vi "Periodic Tasks.vi"(8 "error in":errorcluster) -> ()   [LabVIEW 2023]
doc: "This VI runs in parallel to other tasks. It can contain as many user-defined periodic loops as you need. These can carry out PID or other sorts of timed response."
uses:
  Global odometry.vi
  Global INIT.vi
  <vilib>/Analysis/NI_AAL_Angle.lvlib
  <vilib>/Analysis/coordinate.llb/Wrap Angle (scalar).vi
  <vilib>/Analysis/coordinate.llb/Angle Units.ctl
  <vilib>/Analysis/coordinate.llb/Angle Range (Degree).ctl
  ctrl defs/ctrl DRIVER target assist.ctl
  <vilib>/Rock Robotics/WPI/DriverStation/WPI_DriverStationAllianceInfo.ctl
  ctrl defs/ctrl DRIVING FRAME selector.ctl
  ctrl defs/ctrl pivot select.ctl
  ctrl defs/ctrl driver input.ctl
  ctrl defs/ctrl FRONT FACE selector.ctl
  ctrl defs/ctrl XY coord.ctl
  ctrl defs/ctrl LIMELIGHT STREAM selector.ctl
  ctrl defs/ctrl LIMELIGHT CAMMODE selector.ctl
  ctrl defs/ctrl LIMELIGHT LEDMODE selector.ctl
panel:
  out "LimeLIGHT control":T4 {"stream" items=["standard side-by-side", "PiP Main", "PiP Secondary"]; "camMode" items=["Vision processor", "Driver Camera"]; "ledMode" items=["default to current pipeline", "force off", "force blink", "force on"]}
  out "DRIVER TARGET ASSIST":T5={"ASSIST?"=FALSE, "LOCKED ON?"=FALSE, "DistanceToTarget (in)"=26.235051697949295, "BRNG (deg)"=-2.0}
  out "Continuous Angle":T6
  in  "Update":bool
  out "pivot center":T7 {"Y" format="%.4g"; "X" format="%.4g"}
  out "front face":T8
  out "DRIVER INPUT":T9 {"Jr" format="%.4g"; "theta (rad)" format="%_4f"; "R" format="%.4g"; "Jy" format="%.4g"; "theta (deg)" format="%_4f"; "Jx" format="%.4g"}
  out "select pivot point":T10
  out "drive frame":T11
  out "Alliance":T12
  out "STEER":dbl
  out "DRIVE":dbl
  out "YRPHfH":T13
  out "REAR RIGHT":dbl(knob)
  out "V RR":dbl(knob) scale=-1.0..1.0
  out "FRONT RIGHT":dbl(knob)
  out "V FR":dbl(knob) scale=-1.0..1.0
  out "REAR LEFT":dbl(knob)
  out "V RL":dbl(knob) scale=-1.0..1.0
  out "FRONT LEFT":dbl(knob)
  out "V FL":dbl(knob) scale=-1.0..1.0
  out "Magnetic\nHeadings":cluster{dbl, dbl, dbl}(knob)={0.0, 140.19422999815168, 0.0} scale=0.0..360.0
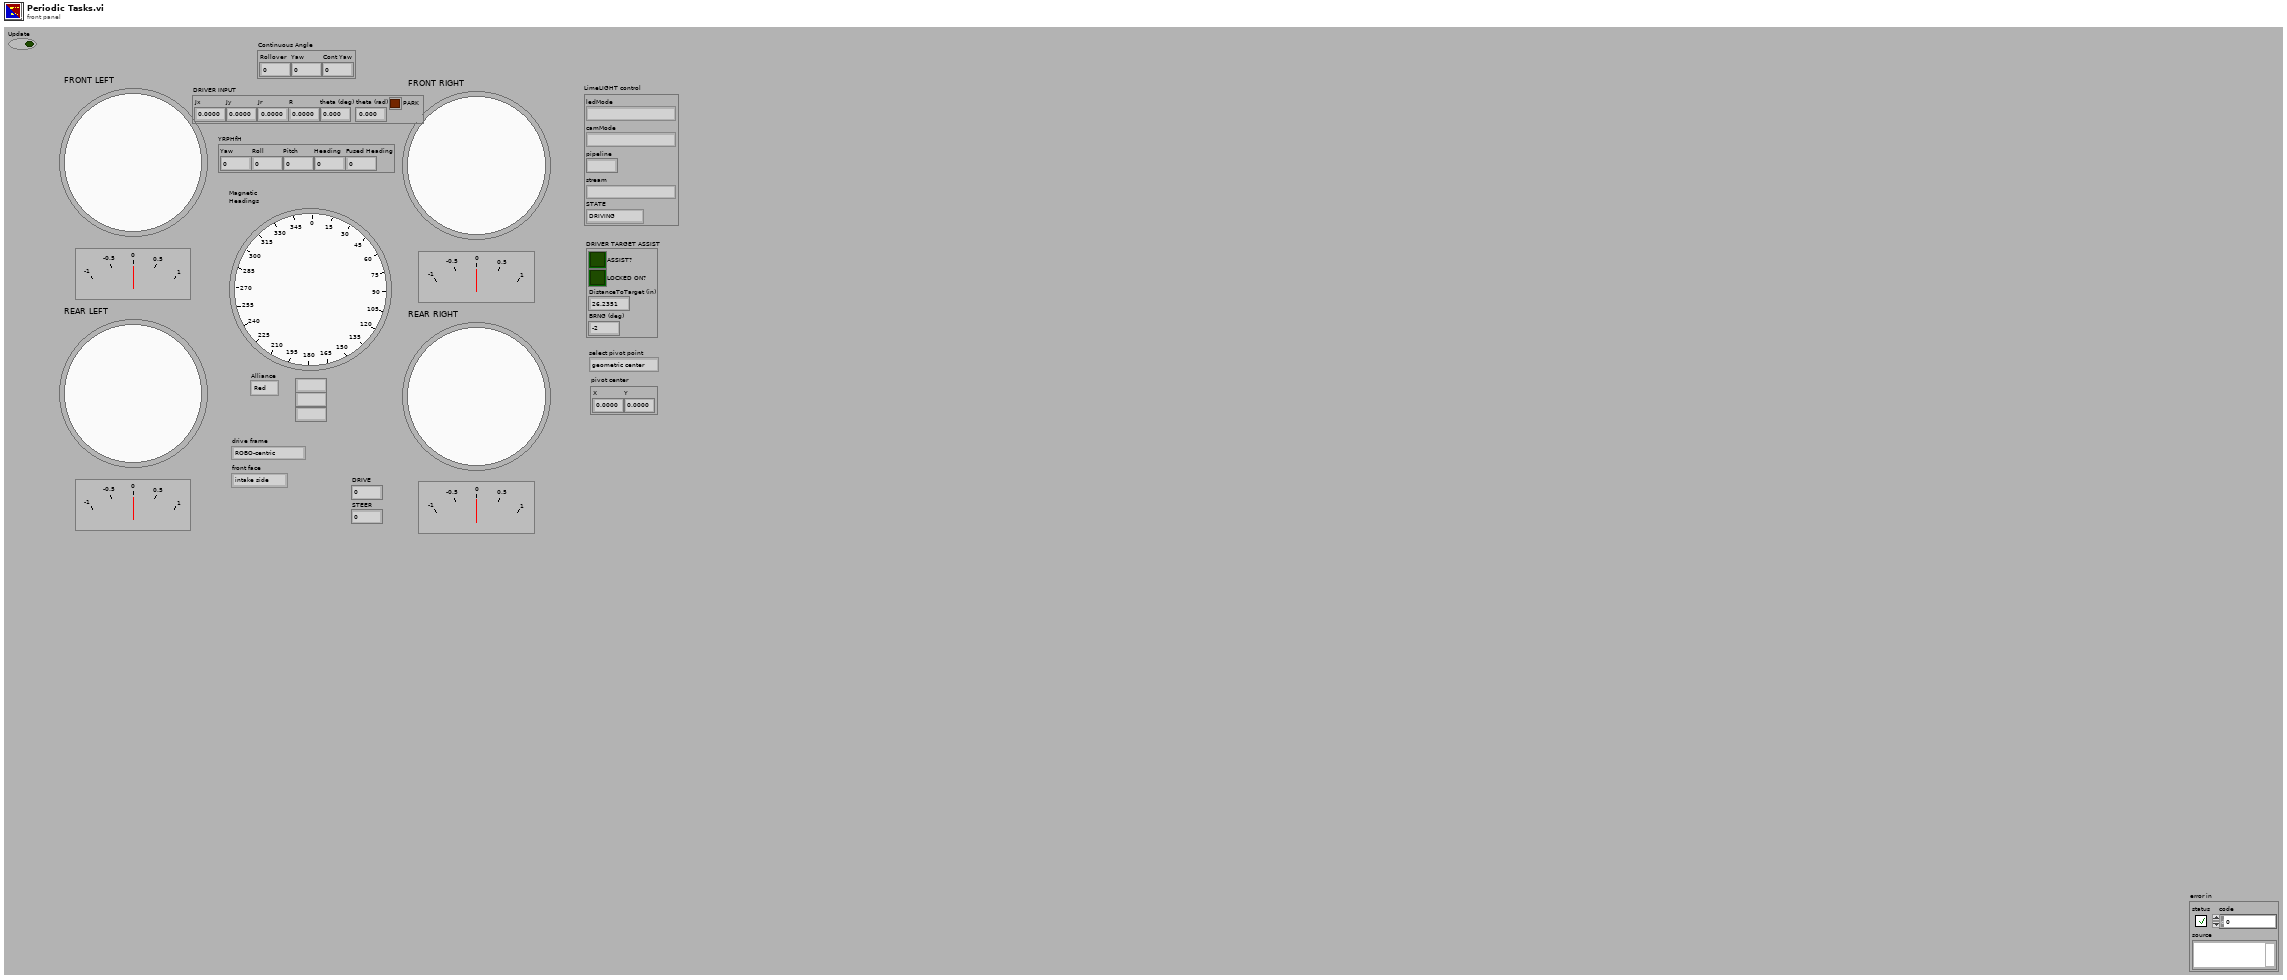
[diagram p1: front panel]
types:
  T1 = typedef "ctrl LIMELIGHT STREAM selector.ctl" = u16
  T2 = typedef "ctrl LIMELIGHT CAMMODE selector.ctl" = u16
  T3 = typedef "ctrl LIMELIGHT LEDMODE selector.ctl" = u16
  T4 = cluster{"stream":T1, "pipeline":u16, "camMode":T2, "ledMode":T3, "STATE":enum16{"DRIVING", "LOOKING for NOTE", "HAVE NOTE"}}
  T5 = typedef "ctrl DRIVER target assist.ctl" = cluster{"ASSIST?":bool, "LOCKED ON?":bool, "DistanceToTarget (in)":dbl, "BRNG (deg)":dbl}
  T6 = cluster{"Rollover":dbl, "Yaw":dbl, "Cont Yaw":dbl}
  T7 = typedef "ctrl XY coord.ctl" = cluster{"X":dbl, "Y":dbl}
  T8 = typedef "ctrl FRONT FACE selector.ctl" = enum16{"intake side", "shooter side"}
  T9 = typedef "ctrl driver input.ctl" = cluster{"Jx":dbl, "Jy":dbl, "Jr ":dbl, "R":dbl, "theta (deg)":dbl, "theta (rad)":dbl, "PARK":bool}
  T10 = typedef "ctrl pivot select.ctl" = enum16{"geometric center", "CG", "FL", "FR", "RR", "RL", "other"}
  T11 = typedef "ctrl DRIVING FRAME selector.ctl" = enum16{"ROBO-centric", "FLD-centric"}
  T12 = typedef "WPI_DriverStationAllianceInfo.ctl" = enum16{"Red", "Blue", "Invalid"}
  T13 = cluster{"Yaw":dbl, "Roll":dbl, "Pitch":dbl, "Heading":dbl, "Fused Heading":dbl}
  T14 = typedef "ctrl LED init.ctl" = cluster{"PWM Channel":T15, "refnum name":string, "#LEDS":T16, "initial output":dbl, "stack name":string, "Installed?":bool, "pattern":T17}
  T15 = typedef "FPGA_DIOPWMChannel.ctl" = enum8{"PWM 0", "PWM 1", "PWM 2", "PWM 3", "PWM 4", "PWM 5", "PWM 6", "PWM 7", "PWM 8", "PWM 9", "PWM MXP 0", "PWM MXP 1", "PWM MXP 2", "PWM MXP 3", "PWM MXP 4", "PWM MXP 5", "PWM MXP 6", "PWM MXP 7", "PWM MXP 8", "PWM MXP 9", "Invalid"}
  T16 = typedef "ctrl number of LEDs.ctl" = u16
  T17 = typedef "ctrl LED PATTERNS.ctl" = u16
  T18 = typedef "ctrl DIO.ctl" = cluster{"description":string, "Installed?":bool, "DIOChannel":T19, "refnum name":string}
  T19 = typedef "FPGA_DIOChannel.ctl" = enum8{"DIO 0", "DIO 1", "DIO 2", "DIO 3", "DIO 4", "DIO 5", "DIO 6", "DIO 7", "DIO 8", "DIO 9", "DIO MXP 0", "DIO MXP 1", "DIO MXP 2", "DIO MXP 3", "DIO MXP 4", "DIO MXP 5", "DIO MXP 6", "DIO MXP 7", "DIO MXP 8", "DIO MXP 9", "DIO MXP 10", "DIO MXP 11", "DIO MXP 12", "DIO MXP 13", "DIO MXP 14", "DIO MXP 15", "SPI Port CS1", "SPI Port CS2", "SPI Port CS3", "SPI Port MISO", "SPI Port MOSI", "Invalid"}
  T20 = typedef "ctrl LIMELIGHT initialize.ctl" = cluster{"Installed?":bool, "pose":cluster{"X":dbl, "Y":dbl, "Z":dbl, "angle to horizon":dbl, "tx angle offset":dbl}}
  T21 = typedef "WPI_DigitalInputDevRef.ctl" = cluster{"DevStatus":errorcluster, "DIO Channel":T19}
  T22 = typedef "ctrl arm motor.ctl" = cluster{" motor":T23, "limit polarities":T29}
  T23 = typedef "ctrl swerve motor.ctl" = cluster{"description":string, "MOTOR SELECT":T24, "Installed?":bool, "CAN ID":u8, "refnum name":string, "Invert":bool, "Idle Mode":T25, "Current limiting":T26, "MOTOR PIDF coefficients":T27, "gear ratio":dbl}
  T24 = typedef "ctrl MOTOR SELECT.ctl" = i16
  T25 = typedef "Spark MAX Idle Mode.ctl" = enum16{"Coast", "Brake"}
  T26 = typedef "ctrl Spark MAX current limiting.ctl" = cluster{"Linearized":bool, "Free Speed (A)":dbl, "Primay (A)":dbl, "Limit RPM (0)":u32}
  T27 = typedef "ctrl motor PIDF coefficients.ctl" = cluster{"PIDF":cluster{"P Gain":dbl, "I Gain":dbl, "D Gain":dbl, "F Gain":dbl, "I Zone":dbl, "Min Output":dbl, "Max Output":dbl}, "Smart Motion":T28}
  T28 = typedef "Spark MAX Smart Motion Parameters.ctl" = cluster{"Max Velocity":dbl, "Max Acceleration":dbl, "Minimum Velocity Output":dbl, "Allowed Closed Loop Error":dbl}
  T29 = typedef "ctrl limit polarity.ctl" = cluster{"Forward limit":T30, "Reverse limit":T30}
  T30 = typedef "Spark MAX Limit Switch Polarity.ctl" = enum16{"Normally Open", "Normally Closed"}
  T31 = typedef "ctrl solenoid.ctl" = cluster{"description":string, "Installed?":bool, "refnum name":string, "coils":enum16{"Single", "Double"}, "forward channel":T32, "reverse channel":T32, "initial value":T33}
  T32 = typedef "WPI_SolenoidChannel.ctl" = enum8{"Solenoid 0", "Solenoid 1", "Solenoid 2", "Solenoid 3", "Solenoid 4", "Solenoid 5", "Solenoid 6", "Solenoid 7", "Solenoid 8", "Solenoid 9", "Solenoid 10", "Solenoid 11", "Solenoid 12", "Solenoid 13", "Solenoid 14", "Solenoid 15", "Invalid"}
  T33 = typedef "WPI_SolenoidValue.ctl" = enum16{"Off", "On", "Forward", "Reverse"}
  T34 = cluster{"LEFT ARM":cluster{"VBus%":dbl, "LOCK?":bool, "LOCKED":bool}, "RIGHT ARM":cluster{"VBus%":dbl, "LOCK?":bool, "LOCKED":bool}}
  T35 = cluster{"VBus%":dbl, "LOCK?":bool, "LOCKED":bool}
  T36 = typedef "NI_AAL_Angle.lvlib/Angle Range (Degree).ctl" = u16
  T37 = typedef "NI_AAL_Angle.lvlib/Angle Units.ctl" = i32
  T38 = cluster{"Heading":dbl, "MAGNETIC Zero for Blue Alliance (deg)":dbl, "angle out":dbl}
  T39 = typedef "ctrl swerve speeds.ctl" = cluster{"NORMAL":cluster{"DRIVE":dbl, "STEER":dbl}, "TURTLE":cluster{"DRIVE":dbl, "STEER":dbl}, "TURBO":cluster{"DRIVE":dbl, "STEER":dbl}}
  T40 = typedef "WPI_MotorControlDeviceRef.ctl" = cluster{"DeviceStatus":errorcluster, "Type":T41, "PWM":cluster{"PWM Channel":T15, "DeadBand":T42}, "CAN":cluster{"Device Number":u8, "SetOutput VI Ref":variant, "GetOutput VI Ref":variant, "Enable VI Ref":variant, "Disable VI Ref":variant, "Data":variant}, "Invert":bool, "DIO PWM":cluster{"PWM \"Enable\" Channel":T15, "DIOChannel":T19, "PWM Rate":dbl}}
  T41 = typedef "WPI_MotorControlType.ctl" = enum16{"PWM", "CAN", "DIO PWM"}
  T42 = typedef "WPI_PWMDeadband.ctl" = cluster{"Name":string, "maxPositivePwm":i32, "minPositivePwm":i32, "centerPwm":i32, "maxNegativePwm":i32, "minNegativePwm":i32, "angularRange":u16}
  T43 = typedef "CTRE_Phoenix_CANcoder_DeviceRef.ctl" = cluster{"DeviceStatus":errorcluster, "Device Number":u8, "Handle":u64, "UsageFrame":u32, "Library Path":path}
  T44 = cluster{"Driver":T40, "Steer":T40, "Encoder":T43}[]
  T45 = typedef "ctrl DRIVER MODE.ctl" = enum16{"default", "TURTLE", "TURBO"}
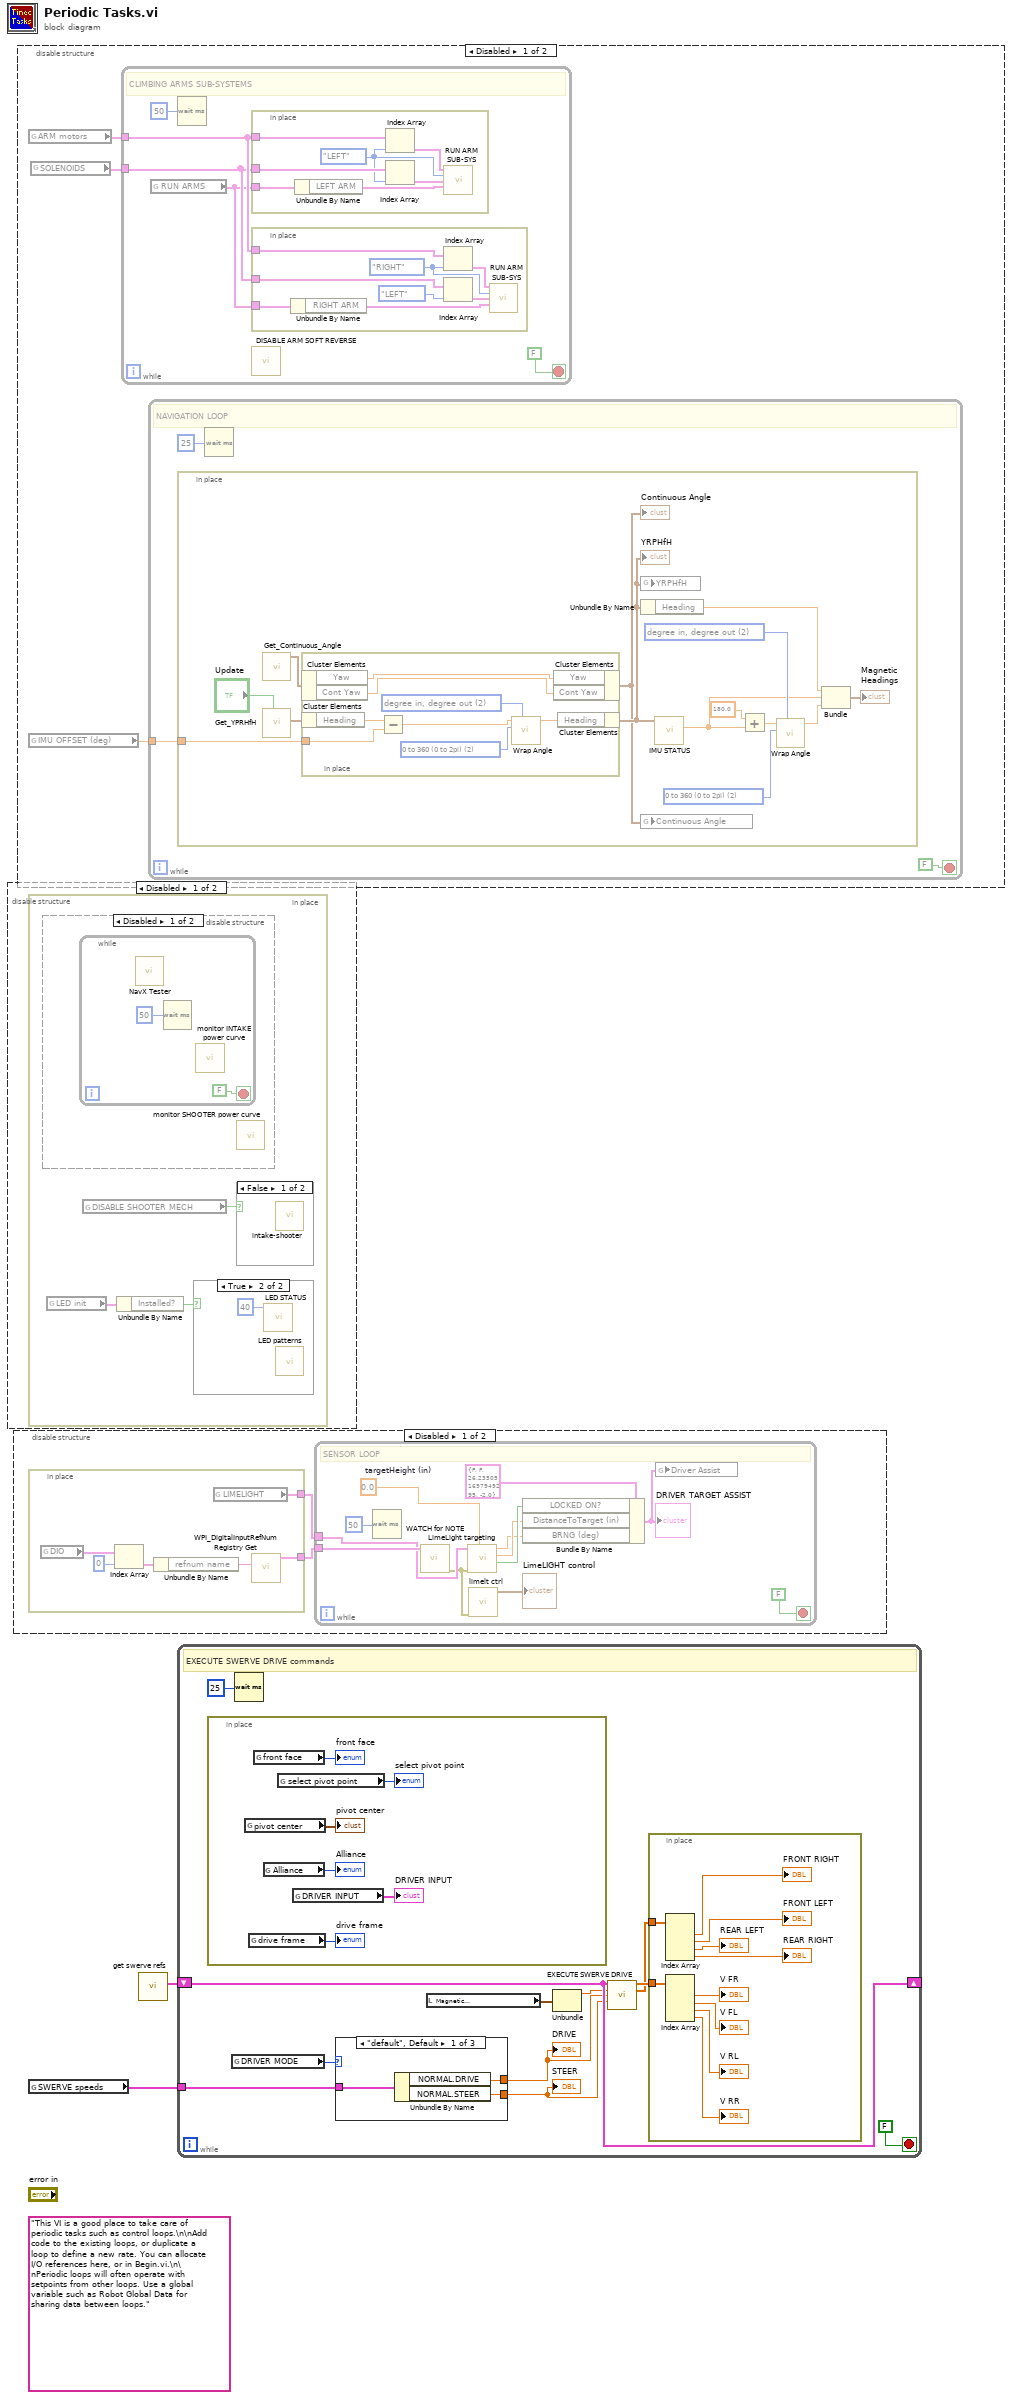
[diagram p0: block diagram]
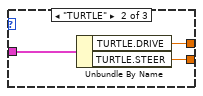
[diagram p8: hidden frame]
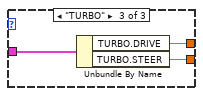
[diagram p9: hidden frame]
diagram:
  (unwired) "This VI is a good place to take care of periodic tasks such as control loops.\n\nAdd code to the existing loops, or duplicate a loop to define a new rate. You can allocate I/O references here, or in Begin.vi.\n\nPeriodic loops will often operate with setpoints from other loops. Use a global variable such as Robot Global Data for sharing data between loops."
  n1 = disable-structure shown="Disabled" {
    frame Disabled {
      n2 = in-place {
        n3 = disable-structure shown="Disabled" {
          frame Disabled {
            n4 = while {
              stop <- FALSE stop-if-true
              n5 = call <vilib>:"NavX Tester.vi"() -> ()  [unwired: 1 in]
              n6 = Wait (ms)(milliseconds to wait=u32 50) -> ()  [unwired: 1 out]
              n7 = call "monitor INTAKE power curve.vi"() -> ()  [unwired: 16 in]
            }
            n8 = call "monitor SHOOTER power curve.vi"() -> ()  [unwired: 16 in]
          }
          frame Enabled {
          }
        }
        n9 = global read "Global INIT.vi" "LED init"() -> (w3:T14)
        n10 = global read "Global INIT.vi" "DISABLE SHOOTER MECH"() -> (w5:bool)
        n11 = Unbundle By Name(w3) -> ("Installed?"=w4:bool)
        n12 = case shown="True" w4 {
          frame False {
          }
          frame True {
            n13 = call "LED STATUS.vi"("LOOP (ms)"=u32 40) -> ()  [unwired: 10 in, 1 out]
            n14 = call "LED patterns.vi"() -> ()  [unwired: 12 in]
          }
        }
        n15 = case shown="False" w5 {
          frame False {
            n16 = call "intake-shooter.vi"() -> ()  [unwired: 12 in]
          }
          frame True {
          }
        }
      }
    }
    frame Enabled {
    }
  }
  n17 = disable-structure shown="Disabled" {
    frame Disabled {
      n18 = in-place {
        in-place-border: [w24] -> w10
        in-place-border: [w23] -> w9
        n19 = global read "Global INIT.vi" "DIO"() -> (w28:T18[])
        n20 = Index Array(array=w28, index=0) -> (element=w26:T18)
        n21 = Unbundle By Name(w26) -> ("refnum name"=w25:string)
        n22 = global read "Global INIT.vi" "LIMELIGHT"() -> (w23:T20)
        n23 = call <vilib>:"WPI_DigitalInputRefNum Registry Get.vi"("refnum name"=w25) -> ("DigitalInputDevRef"=w24:T21)  [unwired: 9 in, 1 out]
      }
      n24 = while {
        tunnel: w10 -> [w22]
        tunnel: w9 -> [w19]
        stop <- FALSE stop-if-true
        w18 = 0.0  # targetHeight (in)
        # "SENSOR LOOP"
        n25 = Wait (ms)(milliseconds to wait=u32 50) -> ()  [unwired: 1 out]
        n26 = call "WATCH for NOTE.vi"("DigitalInputDevRef"=w22) -> ("error out"=w12:errorcluster)  [unwired: 10 in]
        n27 = call "LimeLight targeting.vi"("targetHeight (in)"=w18, "error in (no error)"=w12, "LIMELIGHT pose"=w19) -> ("LOCK?"=w15:bool, "DistanceToTarget"=w14:dbl, "BRNG (deg)"=w13:dbl)  [unwired: 5 in, 1 out]
        n28 = call "limelt ctrl.vi"("error in (no error)"=w12) -> ("LimeLIGHT control"=→"LimeLIGHT control":T4)  [unwired: 9 in, 1 out]
        n29 = Bundle By Name(cluster=T5 {"ASSIST?"=FALSE, "LOCKED ON?"=FALSE, "DistanceToTarget (in)"=26.235051697949295, "BRNG (deg)"=-2.0} ("Driver Assist"), "LOCKED ON?"=w15, "DistanceToTarget (in)"=w14, "BRNG (deg)"=w13) -> (w16:T5)
        "DRIVER TARGET ASSIST" <- w16
        n30 = global write "Global odometry.vi" "Driver Assist"(w16) -> ()
      }
    }
    frame Enabled {
    }
  }
  n31 = disable-structure shown="Disabled" {
    frame Disabled {
      n32 = global read "Global INIT.vi" "ARM motors"() -> (w30:T22[])
      n33 = global read "Global INIT.vi" "IMU OFFSET (deg)"() -> (w29:dbl)
      n34 = global read "Global INIT.vi" "SOLENOIDS"() -> (w31:T31[])
      n35 = while {
        tunnel: w31 -> [w33]
        tunnel: w30 -> [w34]
        stop <- FALSE stop-if-true
        # "CLIMBING ARMS SUB-SYSTEMS"
        n36 = global read "Global odometry.vi" "RUN ARMS"() -> (w32:T34)
        n37 = Wait (ms)(milliseconds to wait=u32 50) -> ()  [unwired: 1 out]
        n38 = in-place {
          in-place-border: w34 -> [w50]
          in-place-border: w33 -> [w48]
          in-place-border: w32 -> [w47]
          w46 = enum16{"LEFT", "RIGHT"}."LEFT" ("SIDE")
          n39 = Unbundle By Name(w47) -> ("LEFT ARM"=w51:T35)
          n40 = Index Array(array=w50, index=w46) -> (element=w49:T22)
          n41 = Index Array(array=w48, index=w46) -> (element=w45:T31)
          n42 = call "RUN ARM SUB-SYS.vi"("ARM motor"=w49, "SIDE"=w46, "SOLENOID"=w45, "ARM"=w51) -> ()  [unwired: 12 in]
        }
        n43 = in-place {
          in-place-border: w34 -> [w43]
          in-place-border: w33 -> [w41]
          in-place-border: w32 -> [w40]
          w39 = enum16{"LEFT", "RIGHT"}."RIGHT" ("SIDE")
          n44 = Unbundle By Name(w40) -> ("RIGHT ARM"=w44:T35)
          n45 = Index Array(array=w43, index=w39) -> (element=w42:T22)
          n46 = Index Array(array=w41, index=enum16{"LEFT", "RIGHT"}."LEFT" ("SIDE")) -> (element=w38:T31)
          n47 = call "RUN ARM SUB-SYS.vi"("ARM motor"=w42, "SIDE"=w39, "SOLENOID"=w38, "ARM"=w44) -> ()  [unwired: 12 in]
        }
        n48 = call "DISABLE ARM SOFT REVERSE.vi"() -> ()  [unwired: 12 in]
      }
      n49 = while {
        tunnel: w29 -> [w52]
        stop <- FALSE stop-if-true
        # "NAVIGATION LOOP"
        n50 = in-place {
          in-place-border: w52 -> [w59]
          w65 = T36 2 items=["none", "-180 to 180 (-pi to pi)", "0 to 360 (0 to 2pi)"] ("angle range")
          w66 = T37 2 items=["radian in, radian out", "radian in, degree out", "degree in, degree out", "degree in, radian out"] ("angle units")
          n51 = call <vilib>:"Get_Continuous_Angle.vi"() -> ("Continuous Angle"=w56:T6)  [unwired: 11 in]
          n52 = call <vilib>:"Get_YPRHfH.vi"("Update"="Update") -> ("YRPHfH"=w60:T13)  [unwired: 10 in]
          n53 = in-place {
            in-place-border: w59 -> [w71]
            w72 = T36 2 items=["none", "-180 to 180 (-pi to pi)", "0 to 360 (0 to 2pi)"] ("angle range")
            w73 = T37 2 items=["radian in, radian out", "radian in, degree out", "degree in, degree out", "degree in, radian out"] ("angle units")
            n54 = in-place-cluster #1(w56) -> ("Yaw"=w70:dbl, "Cont Yaw"=w69:dbl)
            n55 = in-place-cluster #2(w60) -> ("Heading"=w76:dbl)
            n56 = Subtract(x=w76, y=w71) -> (x-y=w75:dbl)
            n57 = call-poly <vilib>:"Wrap Angle.vi"("angle units"=w73, "angle range"=w72, "angle in"=w75) -> ("angle out"=w74:dbl)  [unwired: 7 in, 1 out]
            n58 = in-place-cluster #1("Yaw"=w70, "Cont Yaw"=w69) -> (w55:T6)
            n59 = in-place-cluster #2("Heading"=w74) -> (w57:T13)
          }
          "YRPHfH" <- w57
          "Continuous Angle" <- w55
          n60 = global write "Global odometry.vi" "YRPHfH"(w57) -> ()
          n61 = Unbundle By Name(w57) -> ("Heading"=w68:dbl)
          n62 = global write "Global odometry.vi" "Continuous Angle"(w55) -> ()
          n63 = call "IMU STATUS.vi"("YRPHfH"=w57) -> ("MAGNETIC Zero for Blue Alliance (deg)"=w63:dbl)  [unwired: 9 in, 1 out]
          n64 = Add(x=180.0, y=w63) -> (x+y=w62:dbl)
          n65 = call-poly <vilib>:"Wrap Angle.vi"("angle units"=w66, "angle range"=w65, "angle in"=w62) -> ("angle out"=w64:dbl)  [unwired: 7 in, 1 out]
          n66 = Bundle("Heading"=w68, "MAGNETIC Zero for Blue Alliance (deg)"=w63, "angle out"=w64) -> (→"Magnetic\nHeadings":T38)  [unwired: 1 in]
        }
        n67 = Wait (ms)(milliseconds to wait=u32 25) -> ()  [unwired: 1 out]
      }
    }
    frame Enabled {
    }
  }
  n68 = global read "Global odometry.vi" "SWERVE speeds"() -> (w1:T39)
  n69 = call "get swerve refs.vi"() -> ("Swerve refs"=w2:T44)  [unwired: 10 in, 1 out]
  n70 = while {
    shift-right: [w84] -> _
    shift-left: w2 -> [w84]
    tunnel: w1 -> [w85]
    stop <- FALSE stop-if-true
    # "EXECUTE SWERVE DRIVE commands"
    n71 = in-place {
      n72 = global read "Global odometry.vi" "pivot center"() -> (→"pivot center":T7)
      n73 = global read "Global odometry.vi" "drive frame"() -> (→"drive frame":T11)
      n74 = global read "Global odometry.vi" "front face"() -> (→"front face":T8)
      n75 = global read "Global odometry.vi" "Alliance"() -> (→"Alliance":T12)
      n76 = global read "Global odometry.vi" "select pivot point"() -> (→"select pivot point":T10)
      n77 = global read "Global odometry.vi" "DRIVER INPUT"() -> (→"DRIVER INPUT":T9)
    }
    n78 = global read "Global odometry.vi" "DRIVER MODE"() -> (w83:T45)
    n79 = Wait (ms)(milliseconds to wait=u32 25) -> ()  [unwired: 1 out]
    n80 = case shown="\"default\", Default" w83 {
      tunnel: w85 -> [w105 w109 w111]
      tunnel: [w106 w108 w112] -> w82
      tunnel: [w104 w107 w110] -> w81
      frame "default", Default {
        n81 = Unbundle By Name(w105) -> ("NORMAL.DRIVE"=w106:dbl, "NORMAL.STEER"=w104:dbl)
      }
      frame "TURTLE" {
        n82 = Unbundle By Name(w109) -> ("TURTLE.DRIVE"=w108:dbl, "TURTLE.STEER"=w107:dbl)
      }
      frame "TURBO" {
        n83 = Unbundle By Name(w111) -> ("TURBO.DRIVE"=w112:dbl, "TURBO.STEER"=w110:dbl)
      }
    }
    "DRIVE" <- w82
    "STEER" <- w81
    n84 = local read "Magnetic\nHeadings"() -> (w80:cluster{dbl, dbl, dbl})
    n85 = Unbundle(w80) -> (w79:dbl)  [unwired: 2 out]
    n86 = call "EXECUTE SWERVE DRIVE.vi"("Swerve refs"=w84, "HEADING"=w79, "DRIVE MAX SPEED"=w82, "STEER MAX speed"=w81) -> ("VELOCITIES"=w78:dbl[], "STEERING\nANGLES (deg)"=w77:dbl[])  [unwired: 10 in]
    n87 = in-place {
      in-place-border: w78 -> [w103]
      in-place-border: w77 -> [w98]
      n88 = Index Array(array=w98) -> (element #1=→"FRONT RIGHT":dbl, element #2=→"FRONT LEFT":dbl, element #3=→"REAR LEFT":dbl, element #4=→"REAR RIGHT":dbl)  [unwired: 4 in]
      n89 = Index Array(array=w103) -> (element #1=→"V FR":dbl, element #2=→"V FL":dbl, element #3=→"V RL":dbl, element #4=→"V RR":dbl)  [unwired: 4 in]
    }
  }
